vi "PERCOBAAN 8 (1).vi"() -> ()   [LabVIEW 2020]
uses:
  <vilib>/Utility/NIReport.llb/Report Type.ctl
  <vilib>/Instr/_visa.llb/VISA Configure Serial Port (Instr).vi
  <vilib>/Utility/NIReport.llb/Append Text Table to Report (wrap).vi
  <vilib>/Utility/NIReport.llb/NI_report.lvclass
  <vilib>/Utility/NIReport.llb/Excel/NI_Excel.lvclass
  <vilib>/Utility/NIReport.llb/NI_ReportGenerationCore.lvlib
panel:
  in  "VISA resource name 2":refnum<visa-resource-name>
  out "Temp 2":dbl(slide) scale=0.0..100.0
  out "Jarak":dbl(slide) scale=0.0..100.0
  out "Humi":dbl(slide) scale=0.0..100.0
  out "Jarak 2":dbl
  out "Jarak 3":dbl(graph)
  out "String 4":string
  out "Temp":dbl
  out "Humi 2":dbl
  out "String 3":string
  out "String":string
  out "String 2":string
  out "Temp 3":dbl(graph)
  out "Humi 3":dbl(graph)
  in  "Stop Button":bool
  in  "report file path":path
  in  "vertical alignment (top)":i32(ring) items=["top", "center", "bottom"]
  in  "horizontal alignment (left)":i32(ring) items=["left", "center", "right"]
  # "Disusun Oleh : \n1. Aldisyah Putra Mahardika   \t\t   (EK-2B/3.32.21.1.02) \n2. Aurelia Alika Putri Widiyanta  \t(EK-2B/3.32.21.1.04) \n3. Fahmi Fathur Rohman     \t\t       (EK-2B/3.32.21.1.08)"
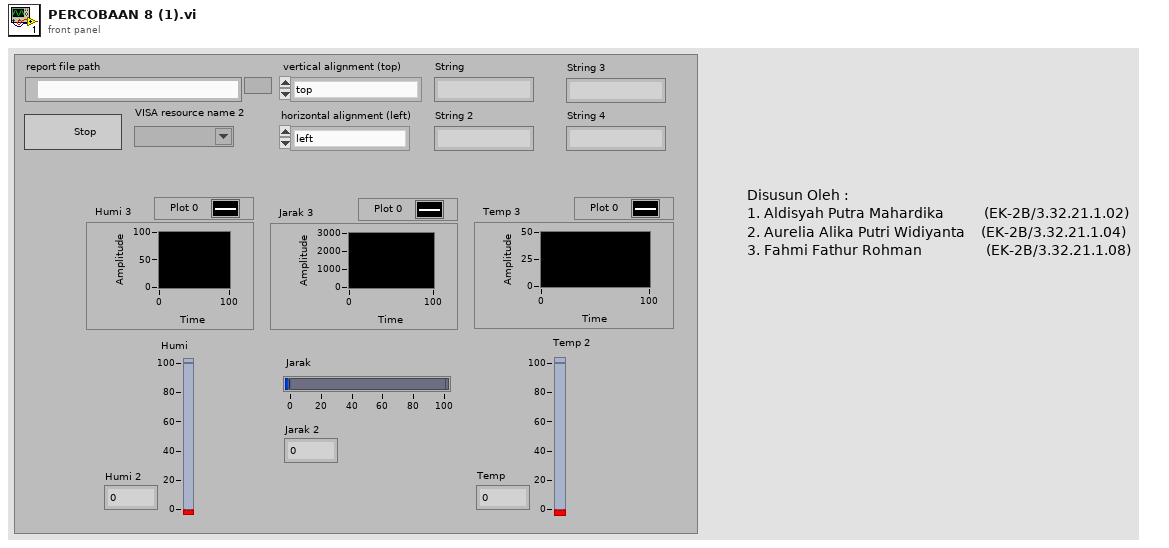
[diagram p1: front panel]
types:
  T1 = typedef "NI_ReportGenerationCore.lvlib/Report Type.ctl" = enum16{"HTML", "Word", "Excel"}
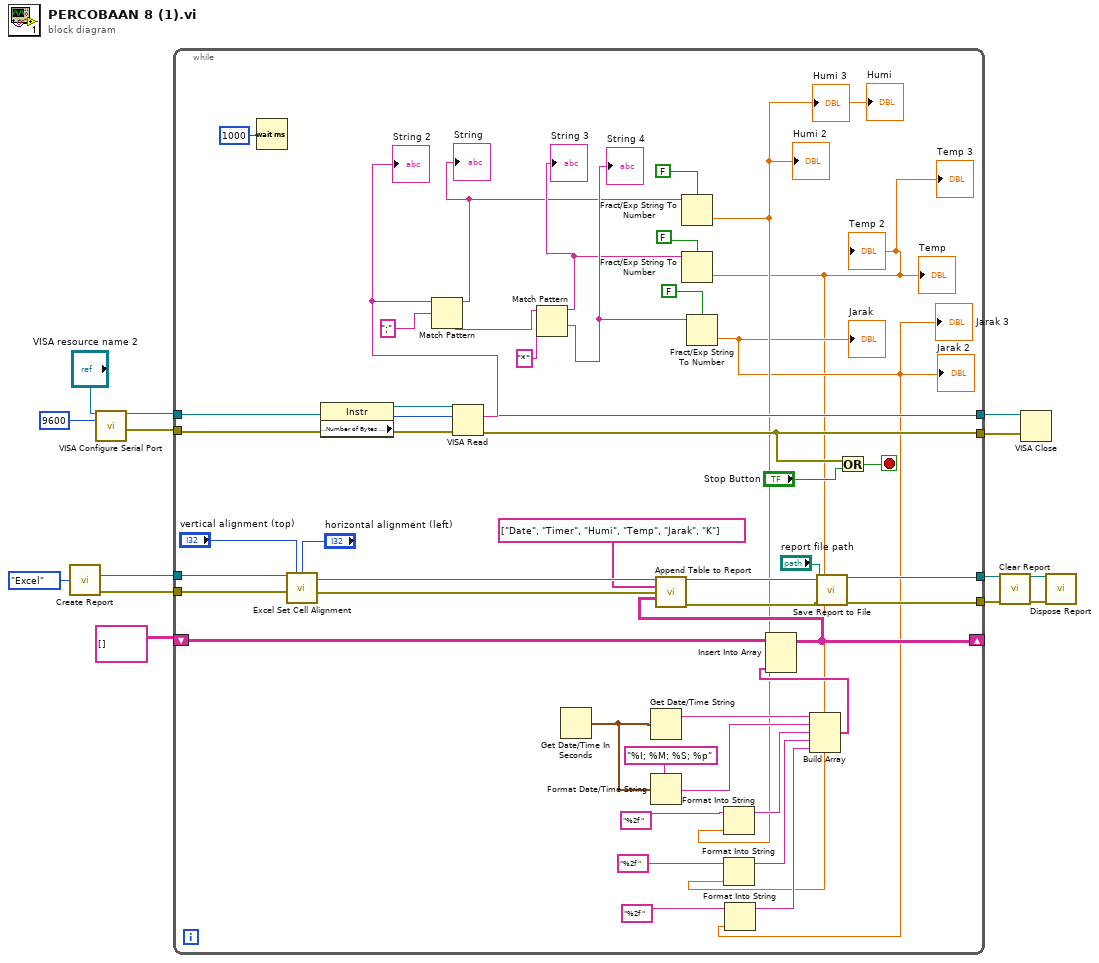
[diagram p0: block diagram]
diagram:
  n1 = call <vilib>:"Create Report.vi"("report type"=Report_Type."Excel") -> ("report out"=w8:refnum<class "NI_report.lvclass">, "error out"=w7:errorcluster)  [unwired: 13 in]
  n2 = call-poly "VISA Configure Serial Port"("VISA resource name"="VISA resource name 2", "baud rate (9600)"=u32 9600) -> ("VISA resource name out"=w4:refnum<visa-resource-name>, "error out"=w3:errorcluster)  [unwired: 12 in]
  n3 = while {
    tunnel: w8 -> [w49]
    tunnel: w7 -> [w48]
    shift-right: [w47] -> _
    shift-left: string[][] [] -> [w46]
    tunnel: [w45] -> w10
    tunnel: [w44] -> w9
    tunnel: w4 -> [w16]
    tunnel: w3 -> [w28]
    tunnel: [w27] -> w1
    tunnel: [w26] -> w2
    stop <- w15 stop-if-true
    n4 = Wait (ms)(milliseconds to wait=u32 1000) -> ()  [unwired: 1 out]
    n5 = call <vilib>:"Excel Set Cell Alignment.vi"("report in"=w49, "vertical alignment (top)"="vertical alignment (top)", "horizontal alignment (left)"="horizontal alignment (left)", "error in (no error)"=w48) -> ("report out"=w56:refnum<class "NI_report.lvclass">, "error out"=w55:errorcluster)  [unwired: 10 in]
    n6 = property class="Instr"(reference=w16, error in=w28) -> (reference out=w42:refnum<visa-resource-name>, error out=w41:errorcluster, "Serial Settings:Number of Bytes at Serial Port"=w32:u32)
    n7 = VISA Read(VISA resource name=w42, byte count=w32, error in (no error)=w41) -> (VISA resource name out=w26:refnum<visa-resource-name>, read buffer=w39:string, error out=w27:errorcluster)  [unwired: 1 out]
    "String 2" <- w39
    n8 = Match Pattern(string=w39, regular expression=";") -> (before substring=w29:string, after substring=w36:string)  [unwired: 1 in, 2 out]
    "String" <- w29
    n9 = Match Pattern(string=w36, regular expression="*") -> (before substring=w30:string, after substring=w34:string)  [unwired: 1 in, 2 out]
    "String 3" <- w30
    "String 4" <- w34
    n10 = Get Date/Time In Seconds() -> (seconds since 1Jan1904=w61:timestamp)
    n11 = Get Date/Time String(seconds (now)=w61) -> (date string=w59:string)  [unwired: 2 in, 1 out]
    n12 = Format Date/Time String(time format string (%c)="%I; %M; %S; %p", seconds (now)=w61) -> (date/time string=w58:string)  [unwired: 1 in]
    n13 = Fract/Exp String To Number(use system decimal point (T)=FALSE, string=w29) -> (number=w19:dbl)  [unwired: 2 in, 1 out]
    "Humi 3" <- w19
    "Humi 2" <- w19
    "Humi" <- w19
    n14 = Fract/Exp String To Number(use system decimal point (T)=FALSE, string=w30) -> (number=w17:dbl)  [unwired: 2 in, 1 out]
    "Temp 3" <- w17
    "Temp" <- w17
    "Temp 2" <- w17
    n15 = Fract/Exp String To Number(use system decimal point (T)=FALSE, string=w34) -> (number=w18:dbl)  [unwired: 2 in, 1 out]
    "Jarak 3" <- w18
    "Jarak 2" <- w18
    "Jarak" <- w18
    n16 = Format Into String(initial string="%2f " ("format string"), w19) -> (resulting string=w25:string)  [unwired: 2 in, 1 out]
    n17 = Format Into String(initial string="%2f ", w17) -> (resulting string=w24:string)  [unwired: 2 in, 1 out]
    n18 = Format Into String(initial string="%2f ", w18) -> (resulting string=w23:string)  [unwired: 2 in, 1 out]
    n19 = Build Array(w59, w58, w25, w24, w23) -> (w57:string[])
    n20 = Insert Into Array(array=w46, new element=w57) -> (w47:string[][])  [unwired: 2 in]
    n21 = call-poly <vilib>:"Append Table to Report.vi"("report in"=w56, "column headers"=string[] ["Date", "Timer", "Humi", "Temp", "Jarak", "K"], "text data"=w47, "error in (no error)"=w55) -> ("report out"=w54:refnum<class "NI_report.lvclass">, "error out"=w53:errorcluster)  [unwired: 8 in, 2 out]
    n22 = call-dynamic "Save Report to File.vi"("report in"=w54, "report file path"="report file path", "error in (no error)"=w53) -> ("report out"=w45:refnum<class "NI_report.lvclass">, "error out"=w44:errorcluster)  [unwired: 11 in]
    n23 = Or(x=w27, y="Stop Button") -> (x .or. y?=w15:bool)
  }
  n24 = call-dynamic "Clear Report.vi"("report in"=w10, "error in (no error)"=w9) -> ("report out"=w12:refnum<class "NI_report.lvclass">, "error out"=w11:errorcluster)  [unwired: 12 in]
  n25 = VISA Close(VISA resource name=w2, error in (no error)=w1) -> ()  [unwired: 1 out]
  n26 = call-dynamic "Dispose Report.vi"("report in"=w12, "error in (no error)"=w11) -> ()  [unwired: 13 in, 1 out]
